vi "TranslationStageDeInitDone.vi"(8 "error in (no error)":errorcluster, 10 "Variant":variant, 11 "Arduino_TranslationStage_UI.lvlib:Arduino_Stepper.lvclass":refnum<class "Arduino_Stepper.lvclass">) -> (0 "error out":errorcluster, 3 "Arduino_TranslationStage_UI.lvlib:Arduino_Stepper.lvclass":refnum<class "Arduino_Stepper.lvclass">)   [LabVIEW 2023, in "Arduino_TranslationStage_UI.lvlib" / "Arduino_Stepper.lvclass"]
uses:
  Arduino_Stepper.lvclass
  Arduino_Stepper.lvclass/Arduino_Stepper.ctl
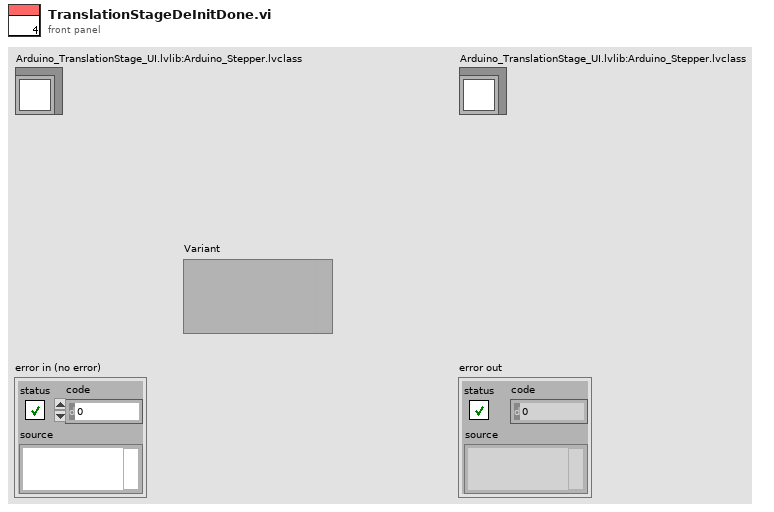
[diagram p1: front panel]
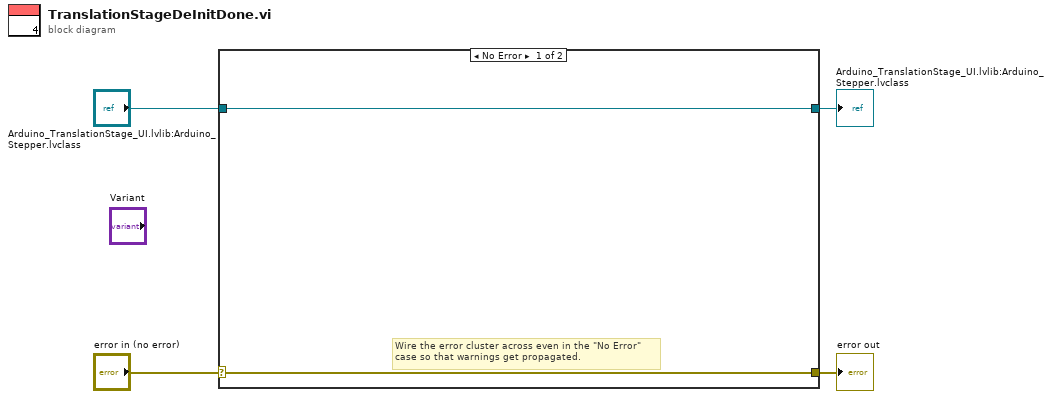
[diagram p0: block diagram]
diagram:
  n1 = case shown="No Error" "error in (no error)" {
    selector: "error in (no error)" -> [w5 w8]
    tunnel: [w5 w8] -> w3
    tunnel: [w6 w7] -> w1
    tunnel: "Arduino_TranslationStage_UI.lvlib:Arduino_Stepper.lvclass" -> [w6 w7]
    frame No Error {
      # "Wire the error cluster across even in the \"No Error\"\ncase so that warnings get propagated."
    }
    frame Error {
    }
  }
  "error out" <- w3
  "Arduino_TranslationStage_UI.lvlib:Arduino_Stepper.lvclass" <- w1
